vi "Read.Lookup.vi"(8 "error in (no error)":errorcluster, 10 "Name":string, 11 "Data Access API in":refnum<class "Data Access API.lvclass">) -> (0 "error out":errorcluster, 2 "Ref":refnum<data-value>, 3 "Data Access API out":refnum<class "Data Access API.lvclass">)   [LabVIEW 2015, in "Data Access API.lvlib" / "Data Access API.lvclass"]
uses:
  Data Access API.lvclass
  Data/Read/Read.lvclass
  Data Access API.lvclass/Data Access API.ctl
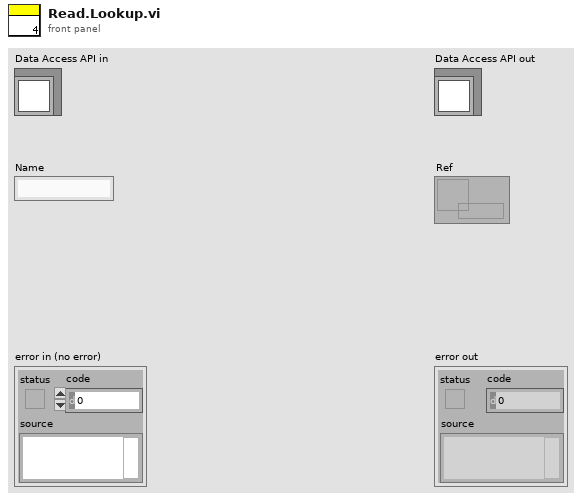
[diagram p1: front panel]
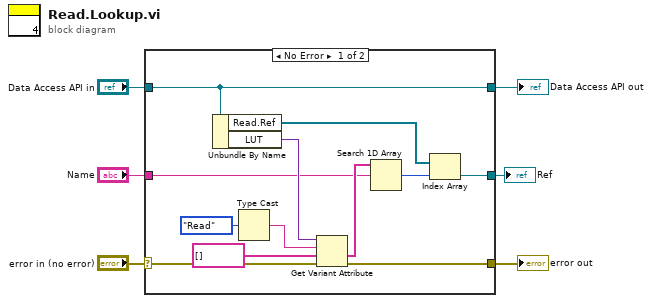
[diagram p0: block diagram]
diagram:
  n1 = case shown="No Error" "error in (no error)" {
    selector: "error in (no error)" -> [w13 w20]
    tunnel: [w12 w20] -> w5
    tunnel: [w18 w19] -> w3
    tunnel: "Data Access API in" -> [w18 w19]
    tunnel: "Name" -> [w10 _]
    tunnel: [w7 _] -> w1
    frame No Error {
      n2 = Unbundle By Name(w18) -> ("Read.Ref"=w8:refnum<data-value>[], "LUT"=w17:variant)
      n3 = Type Cast(x=enum16{"Read", "Write", "ReadWrite"}."Read" ("Type")) -> (*(type *) &x=w15:string)  [unwired: 1 in]
      n4 = Get Variant Attribute(Variant=w17, name=w15, default value (empty Variant)=string[] [], error in=w13) -> (value=w11:string[], error out=w12:errorcluster)  [unwired: 2 out]
      n5 = Search 1D Array(1D array=w11, element=w10) -> (index of element=w9:i32)  [unwired: 1 in]
      n6 = Index Array(array=w8, index=w9) -> (element=w7:refnum<data-value>)
    }
    frame Error {
    }
  }
  "error out" <- w5
  "Data Access API out" <- w3
  "Ref" <- w1
